vi "I2C Main.vi"() -> ()   [LabVIEW 2017]
uses:
  <vilib>/FPGAPlugInAG/cRIO-9035 (Sync)/niLvFpga_Open_cRIO-9035 (Sync).vi
  <vilib>/rvi/interface/common/dynamic/niFpgaDynamicAddResources.vi
  <vilib>/FPGAPlugInAG/Dynamic/niLvFpga_Close_Dynamic.vi
  <vilib>/rvi/interface/nirviOpenFPGA/nirviOpenFPGA.xnode
  FPGA Bitfiles/Pod2_FPGATarget_I2CFPGA_lcZjra3ibCw.lvbitx
  Desktop/I2C Host FPGA/I2C Host FPGA/I2C FPGA.vi
  <vilib>/rvi/interface/nirviCloseFPGA/nirviCloseFPGA.xnode
  <vilib>/IEDriver/SPIandI2C/Host/I2C/I2C Host.lvlib
panel:
  out "error out":errorcluster
  in  "Address Type (7-bit)":enum16{"7-bit", "10-bit"}(ring)
  out "Read Data":u8[](array[numeric])
  in  "Timeout (10 s)":u8=10
  in  "Write Data":u8[](array[numeric])=[80] format="%.0x"
  in  "Clock Rate":u32=1000
  in  "FPGA Clock (40 MHz)":u32=40000000
  in  "Port Number":u8
  in  "Address":u16=25 format="%.0x"
  # "This example demonstrates how to use I2C driver to communicate with I2C device.\nThis example is intentionally broken until you compile this example for a specific target."
  # "Configuration"
  # "Write"
  # "Read"
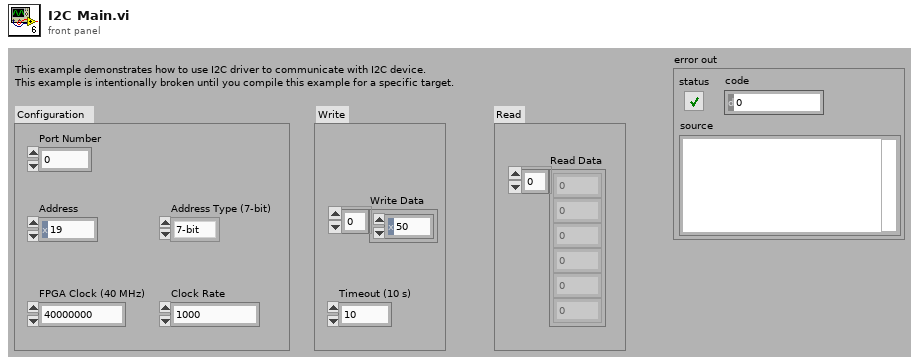
[diagram p1: front panel]
types:
  T1 = cluster{"FPGA VI Reference":refnum<k20>, "Port Number":u8}
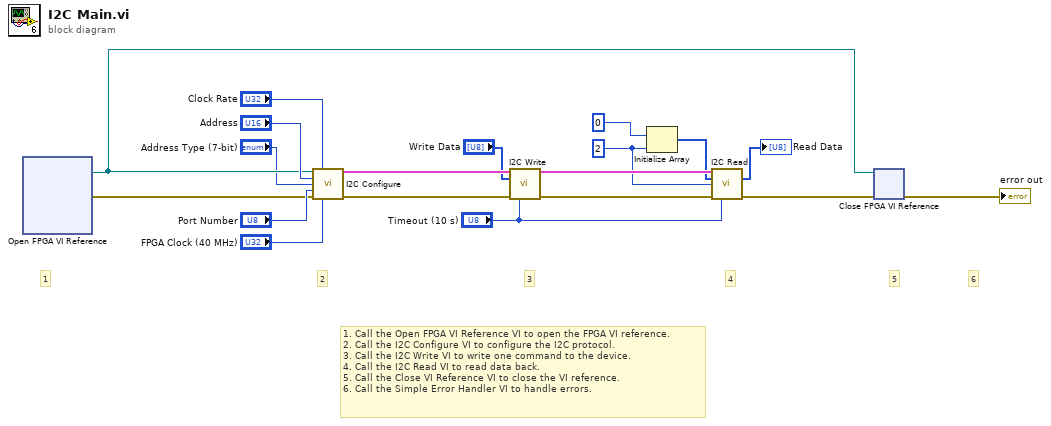
[diagram p0: block diagram]
diagram:
  w7 = u16 2 ("Number of Bytes to Read")
  # "1. Call the Open FPGA VI Reference VI to open the FPGA VI reference.\n2. Call the I2C Configure VI to configure the I2C protocol.\n3. Call the I2C Write VI to write one command to the device.\n4. Call the I2C Read VI to read data back.\n5. Call the Close VI Reference VI to close the VI reference.\n6. Call the Simple Error Handler VI to handle errors."
  # "6"
  # "5"
  # "4"
  # "3"
  # "2"
  # "1"
  n1 = xnode "Open FPGA VI Reference"() -> ("FPGA VI Reference Out"=w2:refnum<k20>, "error out"=w3:errorcluster)  [unwired: 2 in]
  n2 = call <vilib>:"I2C Configure.vi"("FPGA VI Reference"=w2, "Clock Rate"="Clock Rate", "Address"="Address", "Address Type (7-bit)"="Address Type (7-bit)", "Port Number"="Port Number", "error in (no error)"=w3, "FPGA Clock (40 MHz)"="FPGA Clock (40 MHz)") -> ("FPGA Information Out"=w12:T1, "error out"=w19:errorcluster)  [unwired: 7 in]
  n3 = call <vilib>:"I2C Write.vi"("FPGA Information In"=w12, "Data"="Write Data", "error in (no error)"=w19, "Timeout (10 s)"="Timeout (10 s)") -> ("FPGA Information Out"=w11:T1, "error out"=w18:errorcluster)  [unwired: 10 in]
  n4 = Initialize Array(u8 0, w7) -> (w5:u8[])
  n5 = call <vilib>:"I2C Read.vi"("FPGA Information In"=w11, "Input Array"=w5, "Number of Bytes to Read"=w7, "error in (no error)"=w18, "Timeout (10 s)"="Timeout (10 s)") -> ("Data"=→"Read Data":u8[], "error out"=w17:errorcluster)  [unwired: 8 in, 1 out]
  n6 = xnode "Close FPGA VI Reference"("FPGA VI Reference In"=w2, "error in"=w17) -> ("error out"=→"error out":errorcluster)
